vi "Hang Teleop.vi"(10 "axis for motor power":dbl[](array[numeric]), 11 "buttons":bool[](array[boolean])) -> ()   [LabVIEW 2019]
panel:
  out "motor value":dbl
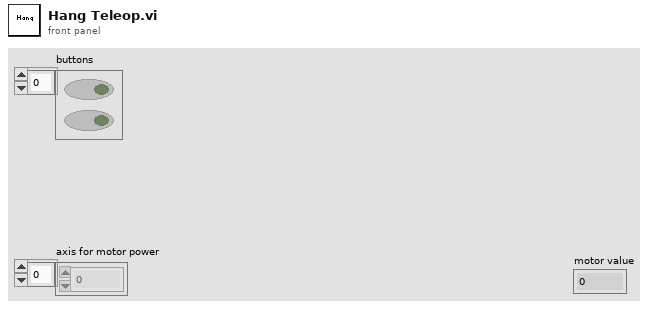
[diagram p1: front panel]
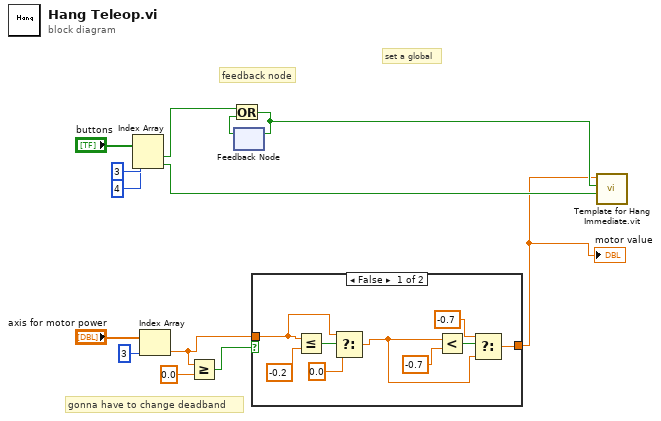
[diagram p0: block diagram]
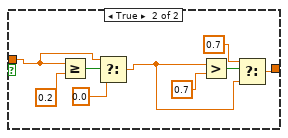
[diagram p2: hidden frame]
diagram:
  # "gonna have to change deadband"
  # "set a global"
  # "feedback node"
  n1 = Index Array(array="buttons", index #1=3 ("index"), index #2=4 ("index")) -> (element #1=w8:bool, element #2=w6:bool)
  n2 = Index Array(array="axis for motor power", index=3) -> (element=w9:dbl)
  n3 = Greater Or Equal?(x=w9, y=0.0) -> (x >= y?=w10:bool)
  n4 = feedback #1() -> (w7:bool)  [unwired: 1 in]
  n5 = Or(x=w8, y=w7) -> (x .or. y?=w5:bool)
  n6 = feedback-in #1(w5) -> ()
  n7 = case shown="False" w10 {
    tunnel: w9 -> [w19 w25]
    tunnel: [w14 w23] -> w1
    frame False {
      n8 = Less Or Equal?(x=w19, y=-0.2) -> (x <= y?=w22:bool)
      n9 = Select(t=w19, s=w22, f=0.0) -> (s? t:f=w15:dbl)
      n10 = Less?(x=w15, y=-0.7) -> (x < y?=w17:bool)
      n11 = Select(t=-0.7, s=w17, f=w15) -> (s? t:f=w14:dbl)
    }
    frame True {
      n12 = Greater Or Equal?(x=w25, y=0.2) -> (x >= y?=w31:bool)
      n13 = Select(t=w25, s=w31, f=0.0) -> (s? t:f=w24:dbl)
      n14 = Greater?(x=w24, y=0.7) -> (0:w27:bool)
      n15 = Select(t=0.7, s=w27, f=w24) -> (s? t:f=w23:dbl)
    }
  }
  "motor value" <- w1
  n16 = call "Template for Hang Immediate.vit"("Ratchet"=w6, "Activation?"=w5, "Motor Power"=w1) -> ()  [unwired: 8 in, 1 out]
